vi "tearDown.vi"(8 "error in":errorcluster, 11 "reference in":refnum<class "Scripting.lvclass">) -> (0 "error out":errorcluster, 3 "reference out":refnum<class "Scripting.lvclass">)   [LabVIEW 2020, in "Scripting.lvclass"]
doc: "tearDown runs after the test method has completed. Use this method to clean up any operations or references that were opened by setUp or the test method. Unit tests should be independent of other unit tests so this VI should ensure that the next test can run in a 'clean' test environment."
uses:
  Scripting.lvclass
  C:/Git/niveristand-custom-device-testing-tools/VeriStandScriptingTestCase/VeriStandScriptingTestCase.lvclass
  niveristand-custom-device-testing-tools/VeriStandScriptingTestCase/VeriStandScriptingTestCase.lvclass
  niveristand-custom-device-testing-tools/VeriStandTestUtilities/VeriStandTestUtilities.lvlib
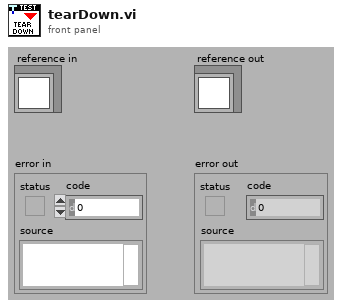
[diagram p1: front panel]
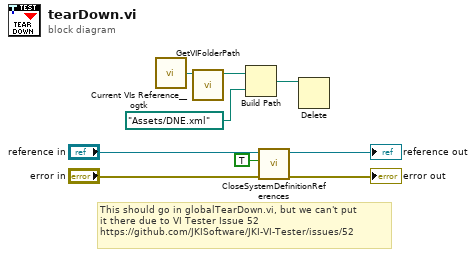
[diagram p0: block diagram]
diagram:
  # "This should go in globalTearDown.vi, but we can't put\nit there due to VI Tester Issue 52\nhttps://github.com/JKISoftware/JKI-VI-Tester/issues/52"
  n1 = call <userlib>:"Current VIs Reference__ogtk.vi"() -> ("Current VI's reference"=w5:refnum<vi>)  [unwired: 5 in]
  n2 = call "GetVIFolderPath.vi"("VI Reference in"=w5) -> ("VI Folder Path out"=w4:path)  [unwired: 9 in, 1 out]
  n3 = Build Path(base path=w4, name or relative path=path "Assets/DNE.xml" ("hardware configuration file path")) -> (appended path=w2:path)
  n4 = call "CloseSystemDefinitionReferences.vi"("error in"="error in", "Delete Sysdef? (F)"=TRUE, "VeriStandScriptingTestCase in"="reference in") -> ("error out"=→"error out":errorcluster, "VeriStandScriptingTestCase out"=→"reference out":refnum<class "Scripting.lvclass">)  [unwired: 7 in]
  n5 = Delete(path (use dialog)=w2) -> ()  [unwired: 4 in, 3 out]
